vi "Arduino Find Home.vi"(5 "Msg Ref":refnum<vi>, 7 "log ref":refnum<file>, 8 "error in":errorcluster, 9 "Homing Parameters":T1, 10 "Motor":i32, 11 "Addr":refnum<visa-resource-name>) -> (0 "error out":errorcluster, 2 "Success":bool, 3 "Log":string)   [LabVIEW 2024, in "FW Arduino Control.lvclass"]
uses:
  FW Arduino Control.lvclass
  Filter Wheel Arduino Homing cluster.ctl
panel:
  in  "Abort":bool
  out "moves":i32
  out "Move distances":i32[](array[numeric])
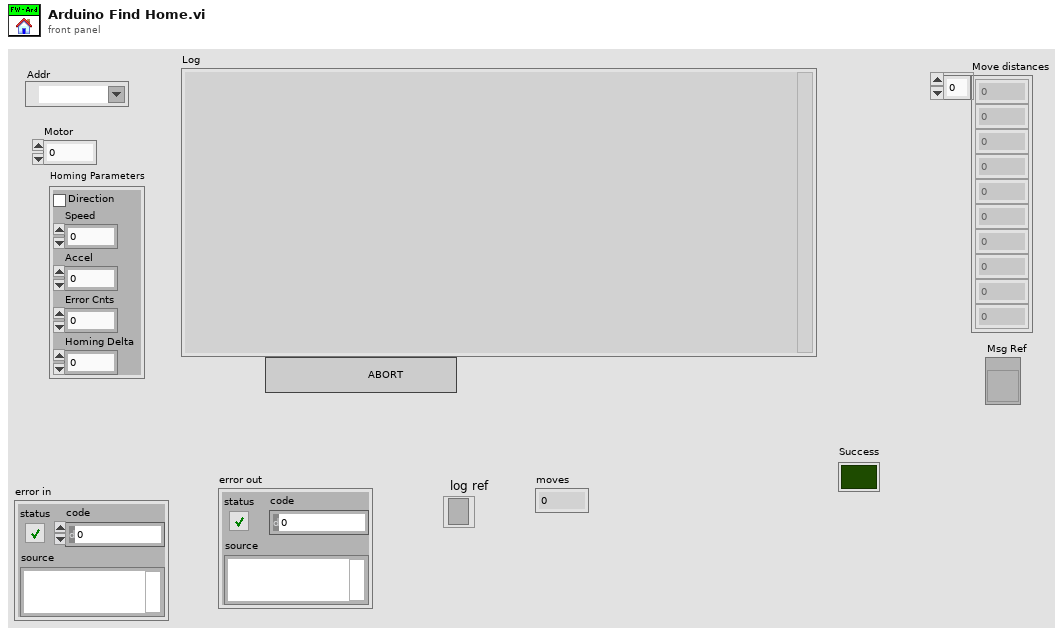
[diagram p1: front panel]
types:
  T1 = typedef "Filter Wheel Arduino Homing cluster.ctl" = cluster{"Direction":bool, "Speed":i32, "Accel":i32, "Error Cnts":i32, "Homing Delta":i32}
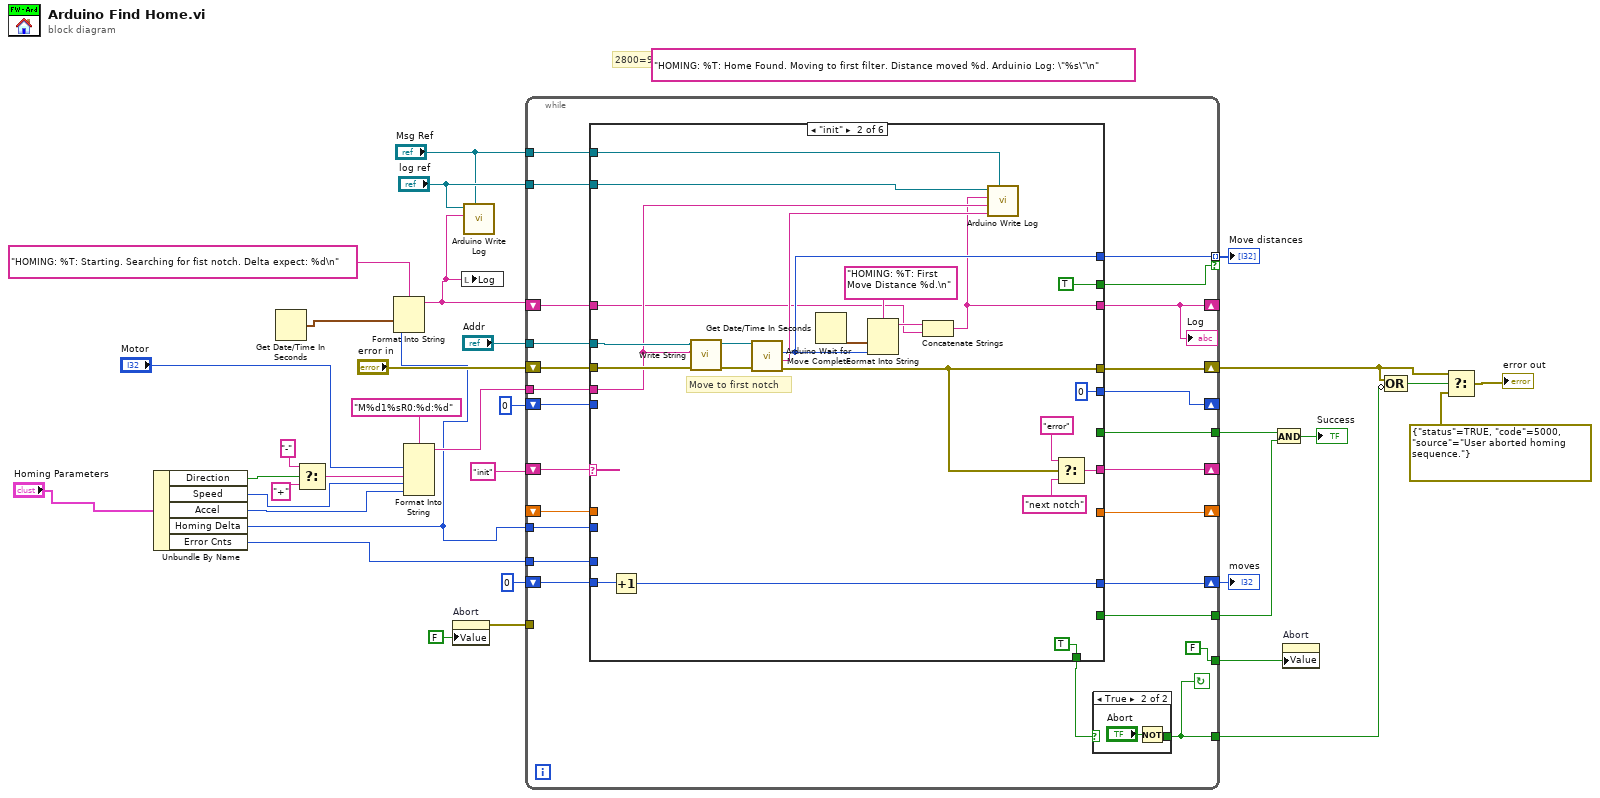
[diagram p0: block diagram]
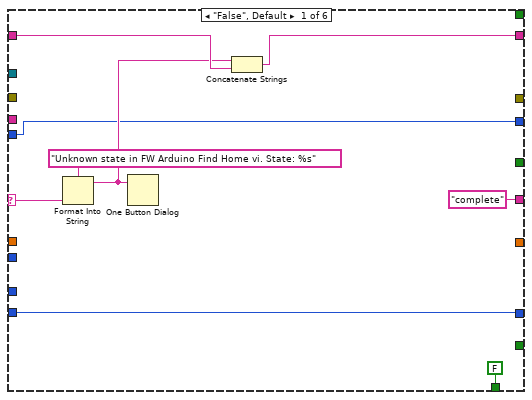
[diagram p3: hidden frame]
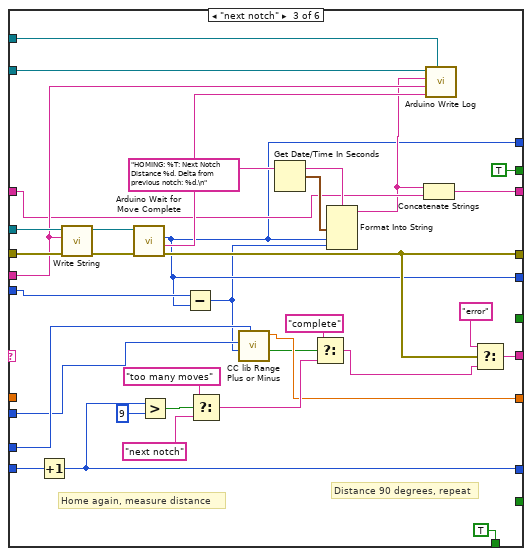
[diagram p4: hidden frame]
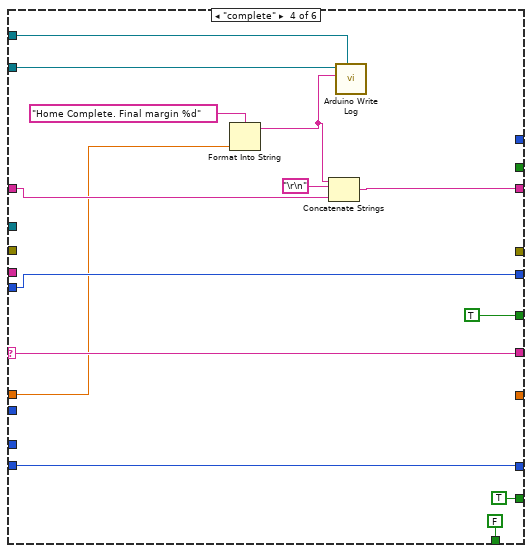
[diagram p5: hidden frame]
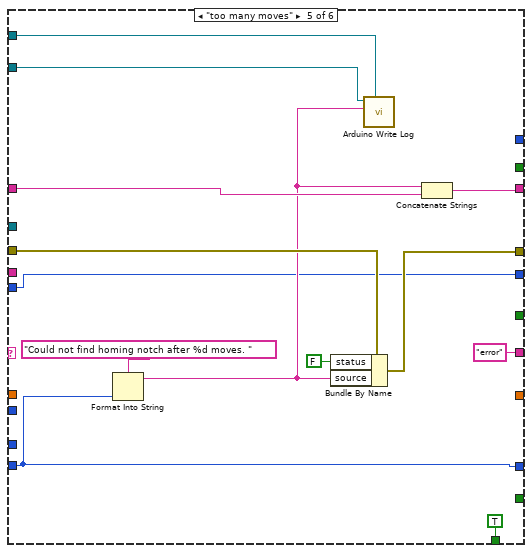
[diagram p6: hidden frame]
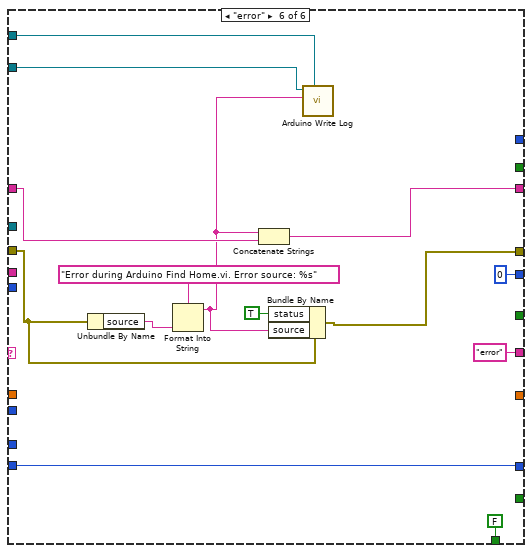
[diagram p7: hidden frame]
diagram:
  (unwired) "HOMING: %T: Home Found. Moving to first filter. Distance moved %d. Arduinio Log: \"%s\"\n" ("format string")
  # "2800=90degrees"
  n1 = Unbundle By Name("Homing Parameters") -> ("Direction"=w27:bool, "Speed"=w26:i32, "Accel"=w25:i32, "Homing Delta"=w1:i32, "Error Cnts"=w16:i32)
  n2 = Get Date/Time In Seconds() -> (seconds since 1Jan1904=w23:timestamp)
  n3 = Select(t="-", s=w27, f="+") -> (s? t:f=w30:string)
  n4 = Format Into String(format string="HOMING: %T: Starting. Searching for fist notch. Delta expect: %d\n", w23, w1) -> (resulting string=w3:string)  [unwired: 2 in, 1 out]
  n5 = Format Into String(format string="M%d1%sR0:%d:%d", "Motor", w30, w26, w25) -> (resulting string=w29:string)  [unwired: 2 in, 1 out]
  n6 = property on="Abort" class="Bool (strict)"("Value"=FALSE ("Abort")) -> (error out=w13:errorcluster)  [unwired: 2 in, 1 out]
  n7 = local write "Log"(w3) -> ()
  n8 = call "Arduino Write Log.vi"("Msg Ref"="Msg Ref", "Message"=w3, "log ref"="log ref") -> ()  [unwired: 9 in]
  n9 = while {
    tunnel: "Addr" -> [w58]
    shift-right: [w59] -> _
    shift-left: "init" -> [w60]
    tunnel: w29 -> [w57]
    shift-right: [w56] -> w9
    shift-left: "error in" -> [w55]
    shift-right: [w42] -> _
    shift-left: w3 -> [w54]
    tunnel: [w53] -> w22
    tunnel: [w52] -> w21 mode=indexing if=w51
    shift-right: [w49] -> w19
    shift-left: 0 -> [w50]
    tunnel: [w48] -> w17
    tunnel: "log ref" -> [w47]
    tunnel: w16 -> [w46]
    tunnel: w1 -> [w45]
    shift-right: [w43] -> _
    shift-left: 0 -> [w44]
    tunnel: w13 -> [_]
    tunnel: [w37] -> w11
    tunnel: [FALSE ("Abort")] -> w6
    shift-right: [w40] -> _
    shift-left: _ -> [w39]
    tunnel: "Msg Ref" -> [w36]
    stop <- w37 continue-if-true
    n10 = case shown="\"init\"" w60 {
      selector: w60 -> [w71 _ _ w142 _ _]
      tunnel: [FALSE TRUE TRUE FALSE TRUE FALSE] -> w38
      tunnel: ["complete" w92 w127 w142 "error" "error"] -> w59
      tunnel: w58 -> [_ w90 w122 _ _ _]
      tunnel: w57 -> [_ w77 w111 _ _ _]
      tunnel: [_ w91 w125 _ w149 w167] -> w56
      tunnel: w55 -> [_ w87 w121 _ w156 w170]
      tunnel: [w66 w75 w109 w140 w148 w159] -> w42
      tunnel: w54 -> [w68 w74 w108 w141 w154 w161]
      tunnel: w45 -> [_ _ w105 _ _ _]
      tunnel: [_ _ _ TRUE _ _] -> w53
      tunnel: [_ w84 w103 _ _ _] -> w52
      tunnel: [_ TRUE TRUE _ _ _] -> w51
      tunnel: w50 -> [w65 w82 w117 w138 w152 w164]
      tunnel: [w65 w81 w115 w138 w152 w164] -> w49
      tunnel: [_ _ _ TRUE _ _] -> w48
      tunnel: w47 -> [_ w80 w112 w136 w147 w163]
      tunnel: w46 -> [_ _ w106 _ _ _]
      tunnel: w44 -> [w64 _ w104 w135 w145 _]
      tunnel: [w64 0 ("distance") w103 w135 w145 0 ("distance")] -> w43
      tunnel: [_ _ w98 _ _ _] -> w40
      tunnel: w39 -> [_ _ _ w132 _ _]
      tunnel: w36 -> [_ w73 w96 w130 w144 w157]
      frame "False", Default {
        n11 = Format Into String(format string="Unknown state in FW Arduino Find Home vi. State: %s", w71) -> (resulting string=w67:string)  [unwired: 2 in, 1 out]
        n12 = One Button Dialog(message=w67) -> ()  [unwired: 1 in, 1 out]
        n13 = Concatenate Strings(w67, w68) -> (w66:string)
      }
      frame "init" {
        # "Move to first notch"
        n14 = Increment(x=w82) -> (x+1=w81:i32)
        n15 = call "Write String.vi"("error in (no error)"=w87, "String"=w77, "VISA resource name"=w90) -> ("error out"=w88:errorcluster, "VISA resource name out"=w89:refnum<visa-resource-name>)  [unwired: 7 in]
        n16 = call "Arduino Wait for Move Complete.vi"("error in (no error)"=w88, "reference"=w89) -> ("error out"=w91:errorcluster, "response"=w78:string, "distance"=w84:i32)  [unwired: 6 in, 1 out]
        n17 = Get Date/Time In Seconds() -> (seconds since 1Jan1904=w85:timestamp)
        n18 = Format Into String(format string="HOMING: %T: First Move Distance %d.\n", w85, w84) -> (resulting string=w79:string)  [unwired: 2 in, 1 out]
        n19 = Concatenate Strings(w79, w74) -> (w75:string)
        n20 = call "Arduino Write Log.vi"("Msg Ref"=w73, "Arduino data"=w78, "Command"=w77, "Message"=w75, "log ref"=w80) -> ()  [unwired: 7 in]
        n21 = Select(t="error", s=w91, f="next notch") -> (s? t:f=w92:string)
      }
      frame "next notch" {
        # "Distance 90 degrees, repeat"
        # "Home again, measure distance"
        n22 = Increment(x=w117) -> (x+1=w115:i32)
        n23 = call "Write String.vi"("error in (no error)"=w121, "String"=w111, "VISA resource name"=w122) -> ("error out"=w124:errorcluster, "VISA resource name out"=w123:refnum<visa-resource-name>)  [unwired: 7 in]
        n24 = call "Arduino Wait for Move Complete.vi"("error in (no error)"=w124, "reference"=w123) -> ("error out"=w125:errorcluster, "response"=w110:string, "distance"=w103:i32)  [unwired: 6 in, 1 out]
        n25 = Greater?(x=w115, y=9) -> (0:w113:bool)
        n26 = Subtract(x=w104, y=w103) -> (x-y=w99:i32)
        n27 = Select(t="too many moves", s=w113, f="next notch") -> (s? t:f=w101:string)
        n28 = call "CC lib Range Plus or Minus.vi"("+/- Range"=w106, "Value"=w99, "Target"=w105) -> ("In Range?"=w97:bool, "margin"=w98:dbl)  [unwired: 6 in, 1 out]
        n29 = Get Date/Time In Seconds() -> (seconds since 1Jan1904=w119:timestamp)
        n30 = Select(t="complete", s=w97, f=w101) -> (s? t:f=w100:string)
        n31 = Format Into String(format string="HOMING: %T: Next Notch Distance %d. Delta from previous notch: %d.\n", w119, w103, w99) -> (resulting string=w107:string)  [unwired: 2 in, 1 out]
        n32 = Concatenate Strings(w107, w108) -> (w109:string)
        n33 = call "Arduino Write Log.vi"("Msg Ref"=w96, "Arduino data"=w110, "Command"=w111, "Message"=w107, "log ref"=w112) -> ()  [unwired: 7 in]
        n34 = Select(t="error", s=w125, f=w100) -> (s? t:f=w127:string)
      }
      frame "complete" {
        n35 = Format Into String(format string="Home Complete. Final margin %d" ("string"), w132) -> (resulting string=w131:string)  [unwired: 2 in, 1 out]
        n36 = Concatenate Strings(w131, "\r\n", w141) -> (w140:string)
        n37 = call "Arduino Write Log.vi"("Msg Ref"=w130, "Message"=w131, "log ref"=w136) -> ()  [unwired: 9 in]
      }
      frame "too many moves" {
        n38 = Format Into String(format string="Could not find homing notch after %d moves. " ("source"), w152) -> (resulting string=w146:string)  [unwired: 2 in, 1 out]
        n39 = Bundle By Name(cluster=w156, "status"=FALSE, "source"=w146) -> (w149:errorcluster)
        n40 = call "Arduino Write Log.vi"("Msg Ref"=w144, "Message"=w146, "log ref"=w147) -> ()  [unwired: 9 in]
        n41 = Concatenate Strings(w146, w154) -> (w148:string)
      }
      frame "error" {
        n42 = Unbundle By Name(w170) -> ("source"=w169:string)
        n43 = Format Into String(format string="Error during Arduino Find Home.vi. Error source: %s", w169) -> (resulting string=w160:string)  [unwired: 2 in, 1 out]
        n44 = Concatenate Strings(w160, w161) -> (w159:string)
        n45 = Bundle By Name(cluster=w170, "status"=TRUE, "source"=w160) -> (w167:errorcluster)
        n46 = call "Arduino Write Log.vi"("Msg Ref"=w157, "Message"=w160, "log ref"=w163) -> ()  [unwired: 9 in]
      }
    }
    "Log" <- w42
    n47 = case shown="True" w38 {
      selector: w38 -> [w61 _]
      tunnel: [w61 w62] -> w37
      frame False {
      }
      frame True {
        n48 = Not(x="Abort") -> (.not. x?=w62:bool)
      }
    }
  }
  "Move distances" <- w21
  "moves" <- w19
  n49 = And(x=w22, y=w17) -> (x .and. y?=→"Success":bool)
  n50 = property on="Abort" class="Bool (strict)"("Value"=w6) -> ()  [unwired: 2 in, 2 out]
  n51 = Compound Arithmetic op=OR(w9, invert w11) -> (w10:bool)
  n52 = Select(t=w9, s=w10, f=errorcluster {"status"=TRUE, "code"=5000, "source"="User aborted homing sequence."}) -> (s? t:f=→"error out":errorcluster)
